vi "CreateBufferSrcDst.vi"(2 "Buffer Src Name":string, 3 "Buffer Dst Name":string, 5 "Error IN":errorcluster) -> (16 "Image Src Result":T1, 17 "Image Dst Result":T1, 19 "Error OUT":errorcluster)   [LabVIEW 2018]
doc: "It creates and return two buffers that reserve memory for two images (one source image and one destination image). Only, it receives two Strings with the desired name for each buffer."
uses:
  <vilib>/vision/Image Controls.llb/IMAQ Image.ctl
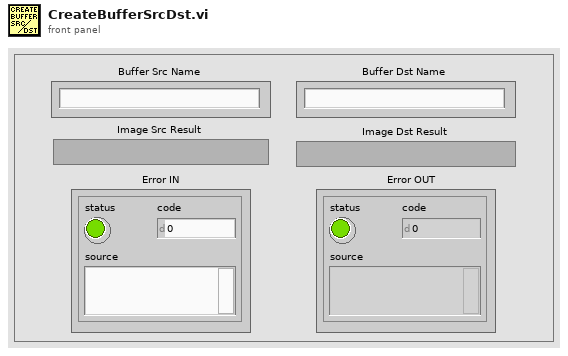
[diagram p1: front panel]
types:
  T1 = typedef "IMAQ Image.ctl" = refnum<image>
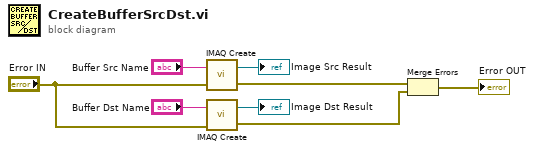
[diagram p0: block diagram]
diagram:
  n1 = call "IMAQ Create"("Image Name"="Buffer Src Name", "error in (no error)"="Error IN") -> ("New Image"=→"Image Src Result":T1, "error out"=w2:errorcluster)  [unwired: 3 in]
  n2 = call "IMAQ Create"("Image Name"="Buffer Dst Name", "error in (no error)"="Error IN") -> ("New Image"=→"Image Dst Result":T1, "error out"=w4:errorcluster)  [unwired: 3 in]
  n3 = Merge Errors(w2, w4) -> (→"Error OUT":errorcluster)
